vi "ma_sml_Three Finger Peak Search.vi"(2 "FFT Size":i32=512, 3 "window length":i32=512, 4 "window":u16(ring) items=["Rectangle"=0, "Hanning"=1, "Hamming"=2, "Blackman-Harris"=3, "Exact Blackman"=4, "Blackman"=5, "Flat Top"=6, "4 Term B-Harris "=7, "7 Term B-Harris"=8, "Low Sidelobe"=9, "Blackman Nuttall"=11, "Triangle"=30, "Bartlett-Hanning"=31, "Bohman"=32, "Parzen"=33, "Welch"=34, "Kaiser"=60, "Dolph-Chebyshev"=61, "Gaussian"=62], 5 "three fingers":dbl[](array[numeric]) format="%.6e") -> (0 "freq":dbl format="%.6f", 1 "amplitude":dbl format="%.2f")   [LabVIEW 2020, in "NI_MAPro.lvlib"]
uses:
  NI_MAPro.lvlib
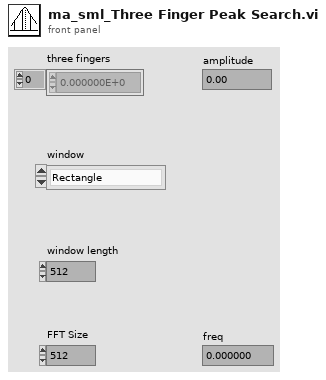
[diagram p1: front panel]
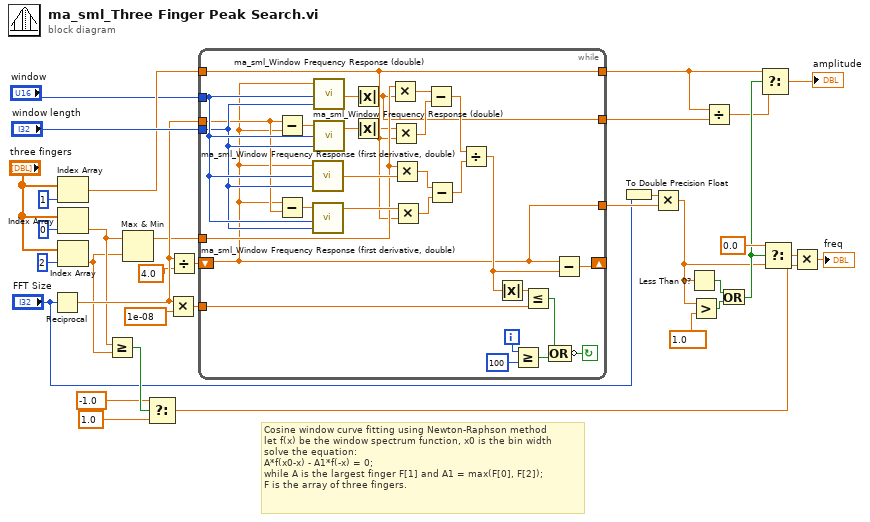
[diagram p0: block diagram]
diagram:
  # "Cosine window curve fitting using Newton-Raphson method\nlet f(x) be the window spectrum function, x0 is the bin width\nsolve the equation:\nA*f(x0-x) - A1*f(-x) = 0;\nwhile A is the largest finger F[1] and A1 = max(F[0], F[2]);\nF is the array of three fingers."
  n1 = Reciprocal(x="FFT Size") -> (1/x=w27:dbl)
  n2 = Index Array(array="three fingers", index=1 ("Index")) -> (element=w21:dbl)
  n3 = Index Array(array="three fingers", index=0 ("Index")) -> (element=w3:dbl)
  n4 = Index Array(array="three fingers", index=2 ("Index")) -> (element=w2:dbl)
  n5 = Greater Or Equal?(x=w3, y=w2) -> (x >= y?=w33:bool)
  n6 = Max & Min(x=w3, y=w2) -> (max(x,y)=w4:dbl)  [unwired: 1 out]
  n7 = Select(t=-1.0, s=w33, f=1.0) -> (s? t:f=w9:dbl)
  n8 = Multiply(x=w27, y=1e-08) -> (x*y=w29:dbl)
  n9 = Divide(x=w27, y=4.0) -> (x/y=w28:dbl)
  n10 = while {
    tunnel: [w38] -> w7
    tunnel: [w36] -> w20
    tunnel: [w45] -> w11
    tunnel: w21 -> [w45]
    tunnel: w29 -> [w39]
    tunnel: w4 -> [w48]
    tunnel: w27 -> [w46]
    tunnel: "window length" -> [w49]
    tunnel: "window" -> [w50]
    shift-left: w28 -> [w38]
    shift-right: [w37] -> _
    i -> [w63]
    stop <- w42 continue-if-true
    n11 = Subtract(x=w46, y=w38) -> (x-y=w61:dbl)
    n12 = Subtract(x=w38, y=w46) -> (x-y=w57:dbl)
    n13 = call "ma_sml_Window Frequency Response (first derivative, double).vi"("N (window length)"=w49, "window"=w50, "f(normalized)"=w38) -> ("H'(f)"=w58:dbl)
    n14 = call "ma_sml_Window Frequency Response (first derivative, double).vi"("N (window length)"=w49, "window"=w50, "f(normalized)"=w57) -> ("H'(f)"=w60:dbl)
    n15 = call "ma_sml_Window Frequency Response (double).vi"("N (window length)"=w49, "window"=w50, "f(normalized)"=w38) -> ("H(f)"=w40:cdb)
    n16 = call "ma_sml_Window Frequency Response (double).vi"("N (window length)"=w49, "window"=w50, "f(normalized)"=w61) -> ("H(f)"=w59:cdb)
    n17 = Absolute Value(x=w40) -> (abs(x)=w36:dbl)
    n18 = Absolute Value(x=w59) -> (abs(x)=w35:dbl)
    n19 = Multiply(x=w48, y=w36) -> (x*y=w56:dbl)
    n20 = Multiply(x=w35, y=w45) -> (x*y=w55:dbl)
    n21 = Multiply(x=w48, y=w58) -> (x*y=w54:dbl)
    n22 = Multiply(x=w60, y=w45) -> (x*y=w53:dbl)
    n23 = Subtract(x=w56, y=w55) -> (x-y=w44:dbl)
    n24 = Subtract(x=w54, y=w53) -> (x-y=w52:dbl)
    n25 = Divide(x=w44, y=w52) -> (x/y=w47:dbl)
    n26 = Absolute Value(x=w47) -> (abs(x)=w51:dbl)
    n27 = Greater Or Equal?(x=w63, y=100) -> (x >= y?=w43:bool)
    n28 = Less Or Equal?(x=w51, y=w39) -> (x <= y?=w41:bool)
    n29 = Compound Arithmetic op=OR(w41, w43) -> (invert w42:bool)
    n30 = Subtract(x=w38, y=w47) -> (x-y=w37:dbl)
  }
  n31 = To Double Precision Float(number="FFT Size") -> (double precision float=w6:dbl)
  n32 = Multiply(x=w6, y=w7) -> (x*y=w8:dbl)
  n33 = Less Than 0?(x=w8) -> (x < 0?=w18:bool)
  n34 = Greater?(x=w8, y=1.0) -> (0:w17:bool)
  n35 = Divide(x=w11, y=w20) -> (x/y=w12:dbl)
  n36 = Or(x=w18, y=w17) -> (x .or. y?=w13:bool)
  n37 = Select(t=w11, s=w13, f=w12) -> (s? t:f=→"amplitude":dbl)
  n38 = Select(t=0.0, s=w13, f=w8) -> (s? t:f=w15:dbl)
  n39 = Multiply(x=w15, y=w9) -> (x*y=→"freq":dbl)
